vi "Sandstorm Handler.vi"(9 "Autonomous VI":refnum<vi>, 10 "Match Info":T1={"Autonomous Elapsed Seconds"=0.0, "TeleOp Elapsed Seconds"=0.0, "Disabled Elapsed Seconds"=0.0, "Visited Autonomous"=FALSE, "Visited TeleOp"=FALSE, "Visited Disabled"=FALSE, "Autonomous Settings"={"Autonomous Style"=enum."Independent", "VI Refnum"=refnum}}, 11 "Call Context":T2) -> ()   [LabVIEW 2018]
uses:
  <vilib>/Rock Robotics/WPI/DriverStation/WPI_DriverStationDerivedRobotMode.ctl
  <vilib>/Rock Robotics/WPI/DriverStation/WPI_DriverStationMatch Info.ctl
  Robot Global Data.vi
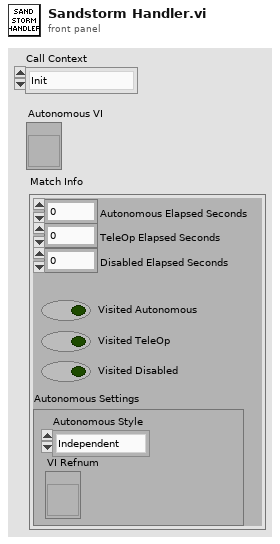
[diagram p1: front panel]
types:
  T1 = typedef "WPI_DriverStationMatch Info.ctl" = cluster{"Autonomous Elapsed Seconds":dbl, "TeleOp Elapsed Seconds":dbl, "Disabled Elapsed Seconds":dbl, "Visited Autonomous":bool, "Visited TeleOp":bool, "Visited Disabled":bool, "Autonomous Settings":cluster{"Autonomous Style":enum16{"Iterative", "Independent"}, "VI Refnum":refnum<vi>}}
  T2 = typedef "WPI_DriverStationDerivedRobotMode.ctl" = enum16{"Init", "Execute", "Stop"}
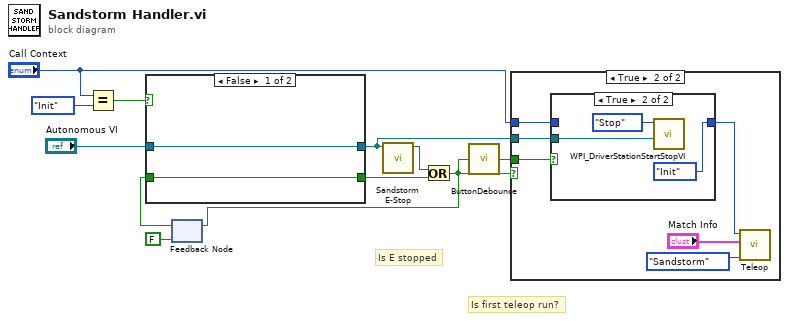
[diagram p0: block diagram]
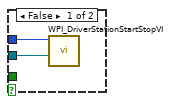
[diagram p2: hidden frame]
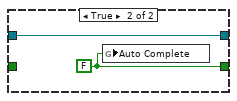
[diagram p4: hidden frame]
diagram:
  # "Is first teleop run?"
  # "Is E stopped"
  n1 = Equal?(x="Call Context", y=WPI_DriverStationDerivedRobotMode."Init") -> (x = y?=w10:bool)
  n2 = feedback #1(FALSE) -> (w8:bool)
  n3 = case shown="False" w10 {
    tunnel: w8 -> [w13 _]
    tunnel: [w13 w15] -> w7
    tunnel: "Autonomous VI" -> [w12 w14]
    tunnel: [w12 w14] -> w1
    frame False {
    }
    frame True {
      w15 = FALSE
      n4 = global write "Robot Global Data.vi" "Auto Complete"(w15) -> ()
    }
  }
  n5 = call "Sandstorm E-Stop.vi"("Autonomous VI"=w1) -> ("Stop Sandstorm"=w3:bool)  [unwired: 10 in]
  n6 = Or(x=w3, y=w7) -> (x .or. y?=w4:bool)
  n7 = feedback-in #1(w4) -> ()
  n8 = call "ButtonDebounce.vi"("Input"=w4) -> ("Output"=w5:bool)
  n9 = case shown="True" w4 {
    tunnel: w1 -> [w17 w21]
    tunnel: "Call Context" -> [w16 w22]
    tunnel: w5 -> [_ w20]
    frame False {
      n10 = call <vilib>:"WPI_DriverStationStartStopVI.vi"("VI in"=w17, "Call Context"=w16) -> ()  [unwired: 10 in]
    }
    frame True {
      n11 = case shown="True" w20 {
        tunnel: [w24 WPI_DriverStationDerivedRobotMode."Init" ("Call Context")] -> w23
        tunnel: w22 -> [w24 _]
        tunnel: w21 -> [_ w25]
        frame False {
        }
        frame True {
          n12 = call <vilib>:"WPI_DriverStationStartStopVI.vi"("VI in"=w25, "Call Context"=WPI_DriverStationDerivedRobotMode."Stop") -> ()  [unwired: 10 in]
        }
      }
      n13 = call "Teleop.vi"("Mode"=enum16{"Sandstorm", "Teleop"}."Sandstorm", "Match Info"="Match Info", "Call Context"=w23) -> ()  [unwired: 9 in]
    }
  }
